vi "Set Impulse Count.vi"(8 "error in (no error)":errorcluster, 10 "Nr of Fit Impulses":i32, 11 "Abstract Fit in":refnum<class "Abstract Fit.lvclass">) -> (0 "error out":errorcluster, 3 "Abstract Fit out":refnum<class "Abstract Fit.lvclass">)   [LabVIEW 2016, in "Abstract Fit.lvclass"]
uses:
  Abstract Fit.lvclass
  Abstract Fit.lvclass/Abstract Fit.ctl
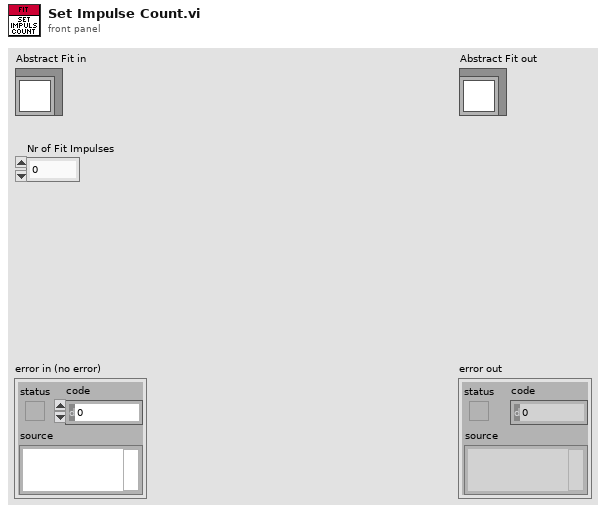
[diagram p1: front panel]
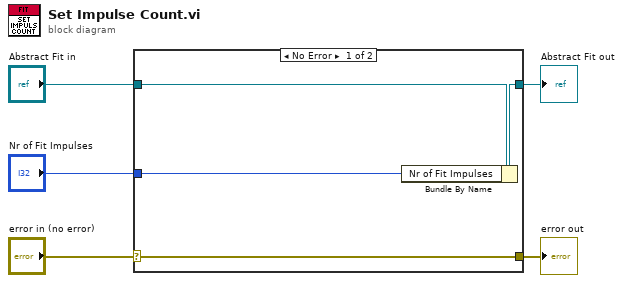
[diagram p0: block diagram]
diagram:
  n1 = case shown="No Error" "error in (no error)" {
    selector: "error in (no error)" -> [w9 w10]
    tunnel: [w9 w10] -> w4
    tunnel: [w7 w11] -> w2
    tunnel: "Abstract Fit in" -> [w8 w11]
    tunnel: "Nr of Fit Impulses" -> [w6 _]
    frame No Error {
      n2 = Bundle By Name(cluster=w8, "Nr of Fit Impulses"=w6) -> (w7:refnum<class "Abstract Fit.lvclass">)
    }
    frame Error {
    }
  }
  "error out" <- w4
  "Abstract Fit out" <- w2
